vi "Append (multiple).vi"(6 "Reset":bool, 8 "error in (no error)":errorcluster, 10 "XY-data (B)":cluster{"X-array":dbl[], "Y-array":dbl[]}[](array[cluster]), 11 "XY-data (A)":cluster{"X-array":dbl[], "Y-array":dbl[]}[](array[cluster])) -> (0 "error out":errorcluster, 3 "XY-data out":cluster{"X-array":dbl[], "Y-array":dbl[]}[](array[cluster]) {"Y-array" format="%.2p"; "X-array" format="%.2p"})   [LabVIEW 2019, in "xy_utilities.lvlib"]
doc: "Append <B>XY-Data B</B> to the end of <B>XY-Data A</B> (similar to Append Waveforms.vi).\n\nWire data to the data input to determine the polymorphic instance to use or manually select the instance."
uses:
  xy_utilities.lvlib
  Append (double array).vi
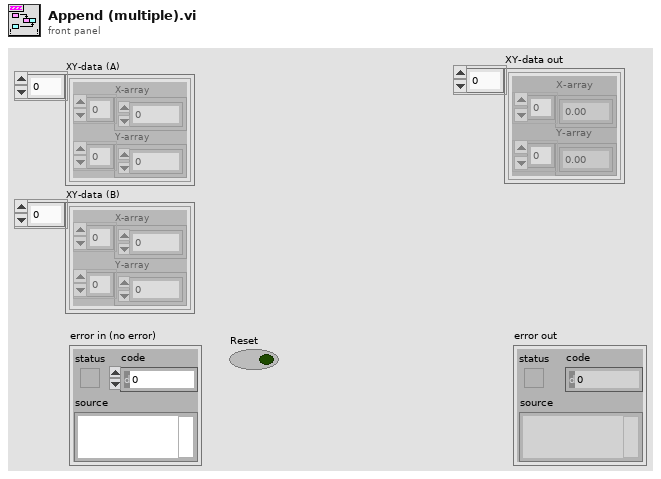
[diagram p1: front panel]
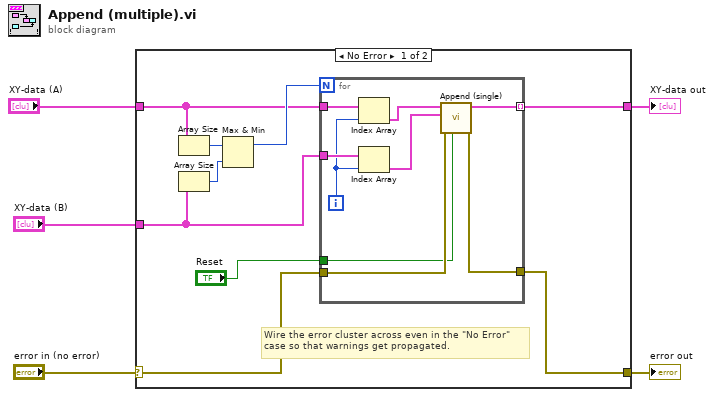
[diagram p0: block diagram]
diagram:
  n1 = case shown="No Error" "error in (no error)" {
    selector: "error in (no error)" -> [w9 w25]
    tunnel: [w8 w25] -> w4
    tunnel: "XY-data (A)" -> [w11 w24]
    tunnel: [w10 w24] -> w3
    tunnel: "XY-data (B)" -> [w6 _]
    frame No Error {
      # "Wire the error cluster across even in the \"No Error\"\ncase so that warnings get propagated."
      n2 = Array Size(array=w11) -> (size(s)=w14:i32)
      n3 = Array Size(array=w6) -> (size(s)=w13:i32)
      n4 = Max & Min(x=w14, y=w13) -> (max(x,y)=w12:i32)  [unwired: 1 out]
      n5 = for {
        N: w12 -> [_]
        tunnel: w11 -> [w23]
        tunnel: w6 -> [w22]
        tunnel: [w20] -> w10 mode=indexing
        tunnel: w9 -> [w19]
        tunnel: [w18] -> w8
        tunnel: "Reset" -> [w16]
        i -> [w17]
        n6 = Index Array(array=w23, index=w17) -> (element=w15:cluster{"X-array":dbl[], "Y-array":dbl[]})
        n7 = Index Array(array=w22, index=w17) -> (element=w21:cluster{"X-array":dbl[], "Y-array":dbl[]})
        n8 = call "Append (single).vi"("Reset"=w16, "error in (no error)"=w19, "XY-data (B)"=w21, "XY-data (A)"=w15) -> ("error out"=w18:errorcluster, "XY-data out"=w20:cluster{"X-array":dbl[], "Y-array":dbl[]})  [unwired: 6 in]
      }
    }
    frame Error {
    }
  }
  "error out" <- w4
  "XY-data out" <- w3
